vi "main.vi"() -> ()   [LabVIEW 2026]
uses:
  StateEnum.ctl
panel:
  in  "VISA resource name":refnum<visa-resource-name>
  out "read buffer":string
  out "error out 2":errorcluster
  in  "error in (no error)":errorcluster
  out "Corriente":dbl(knob) scale=0.0..10.0
  out "Voltaje":dbl(knob) scale=0.0..10.0
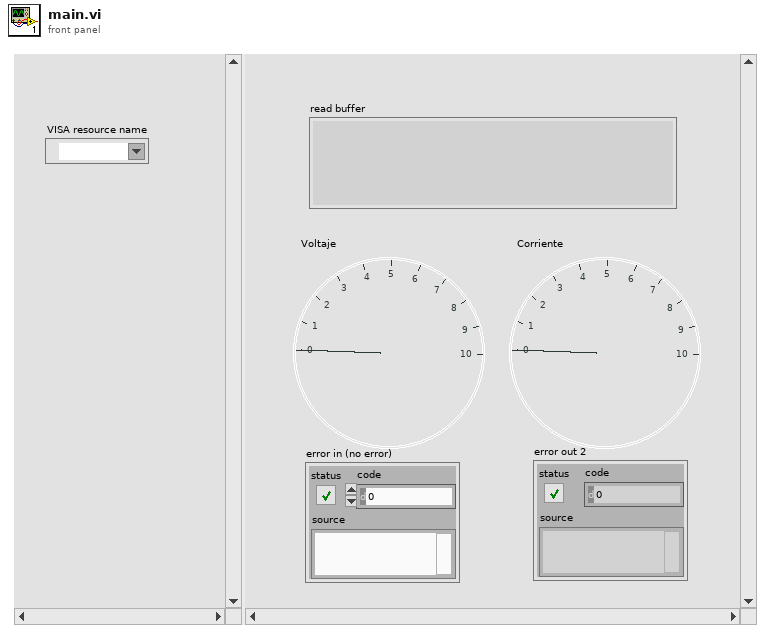
[diagram p1: front panel]
types:
  T1 = typedef "StateEnum.ctl" = enum16{"Idle", "Stop", "Start"}
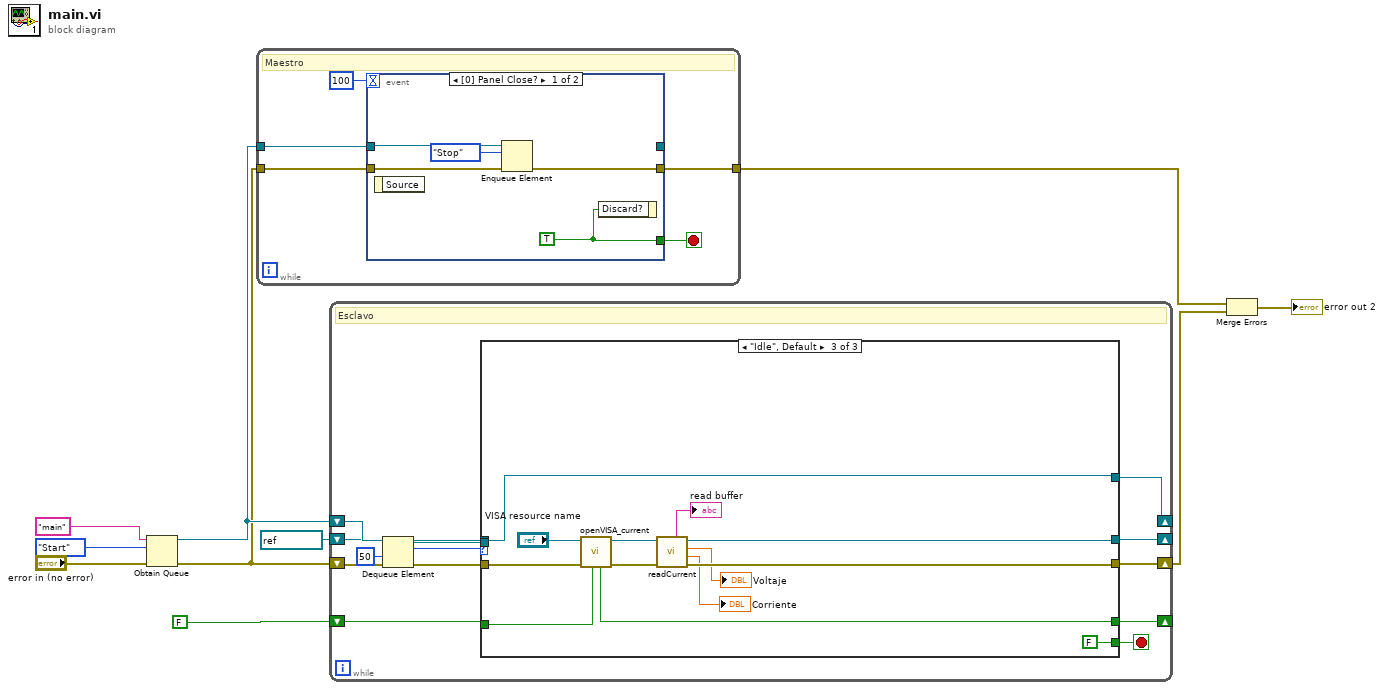
[diagram p0: block diagram]
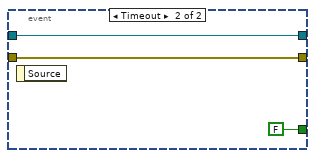
[diagram p2: hidden frame]
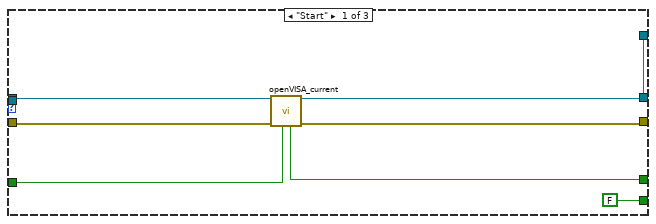
[diagram p3: hidden frame]
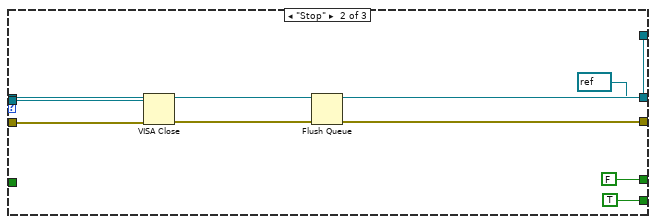
[diagram p4: hidden frame]
diagram:
  n1 = Obtain Queue(name (unnamed)="main", element data type=StateEnum."Start", error in (no error)="error in (no error)") -> (queue out=w7:refnum<queue>, error out=w6:errorcluster)  [unwired: 2 in, 1 out]
  n2 = while {
    tunnel: w6 -> [w13]
    tunnel: [w12] -> w5
    tunnel: w7 -> [w11]
    stop <- w14 stop-if-true
    # "Maestro"
    n3 = event shown="[0] Panel Close?" {
      selector: _ -> [_ _]
      dyn-events: _ -> [_ _]
      timeout: 100 -> [_ _]
      tunnel: [w16 FALSE] -> w14
      tunnel: w13 -> [w19 w23]
      tunnel: [w20 w23] -> w12
      tunnel: w11 -> [w18 w22]
      tunnel: [_ w22] -> _
      event Panel Close? {
        w16 = TRUE
        n4 = event-data() -> ()  [unwired: 1 in, 1 out]
        n5 = Enqueue Element(queue=w18, element=StateEnum."Stop", error in (no error)=w19) -> (error out=w20:errorcluster)  [unwired: 1 in, 2 out]
        n6 = event-data("Discard?"=w16) -> ()  [unwired: 1 in, 1 out]
      }
      event Timeout {
        n7 = event-data() -> ()  [unwired: 1 in, 1 out]
      }
    }
  }
  n8 = while {
    shift-right: [w30] -> w4
    shift-left: w6 -> [w36]
    shift-right: [w29] -> _
    shift-left: refnum<visa-resource-name> "COM6" ("VISA resource name out") -> [w27]
    shift-right: [w25] -> _
    shift-left: FALSE -> [w26]
    shift-right: [w24] -> _
    shift-left: w7 -> [w35]
    stop <- w28 stop-if-true
    # "Esclavo"
    n9 = Dequeue Element(queue=w35, timeout in ms (-1)=50, error in (no error)=w36) -> (queue out=w32:refnum<queue>, element=w31:T1, error out=w33:errorcluster)  [unwired: 1 out]
    n10 = case shown="\"Idle\", Default" w31 {
      tunnel: w33 -> [w42 w49 w63]
      tunnel: w32 -> [w43 w51 w65]
      tunnel: [w37 w52 w64] -> w30
      tunnel: [w41 refnum<visa-resource-name> refnum ("VISA resource name out") w56] -> w29
      tunnel: [FALSE TRUE FALSE] -> w28
      tunnel: w27 -> [w40 w48 _]
      tunnel: [w43 w50 w65] -> w24
      tunnel: w26 -> [w39 _ w55]
      tunnel: [w38 FALSE w54] -> w25
      frame "Start" {
        n11 = call "openVISA_current.vi"("Boolean in"=w39, "error in (no error)"=w42, "VISA Refnum in"=w40) -> ("error out"=w37:errorcluster, "VISA Refnum out"=w41:refnum<visa-resource-name>, "Boolean out"=w38:bool)  [unwired: 6 in]
      }
      frame "Stop" {
        n12 = VISA Close(VISA resource name=w48, error in (no error)=w49) -> (error out=w47:errorcluster)
        n13 = Flush Queue(queue=w51, error in (no error)=w47) -> (queue out=w50:refnum<queue>, error out=w52:errorcluster)  [unwired: 1 out]
      }
      frame "Idle", Default {
        n14 = call "openVISA_current.vi"("Boolean in"=w55, "error in (no error)"=w63, "VISA Refnum in"="VISA resource name") -> ("error out"=w62:errorcluster, "VISA Refnum out"=w59:refnum<visa-resource-name>, "Boolean out"=w54:bool)  [unwired: 6 in]
        n15 = call "readCurrent.vi"("error in (no error)"=w62, "VISA resource name"=w59) -> ("error out"=w64:errorcluster, "Corriente"=→"Corriente":dbl, "Voltaje"=→"Voltaje":dbl, "VISA Refnum out"=w56:refnum<visa-resource-name>, "read buffer"=→"read buffer":string)  [unwired: 3 in]
      }
    }
  }
  n16 = Merge Errors(w5, w4) -> (→"error out 2":errorcluster)
